vi "Statistics.vi"() -> ()   [LabVIEW 2023]
uses:
  <vilib>/Analysis/NI_AALBase.lvlib
panel:
  out "Variance My":dbl[](array[numeric])
  out "STD":dbl[](array[numeric])
  out "Average in row":u64[](array[numeric]) format="%-2.0f"
  out "Deviation by row":i64[][](array[numeric]) format="%.1f"
  out "Max in row":i32[](array[numeric])
  out "Min in row":i32[](array[numeric])
  out "Mean == Average":u64[](array[numeric])
  out "Variance":u64[](array[numeric])
  out "Std Deviation":dbl[](array[numeric]) format="%.4f"
  out "Mean":u64[](array[numeric])
  out "2D Double Array":i32[][](array[numeric])
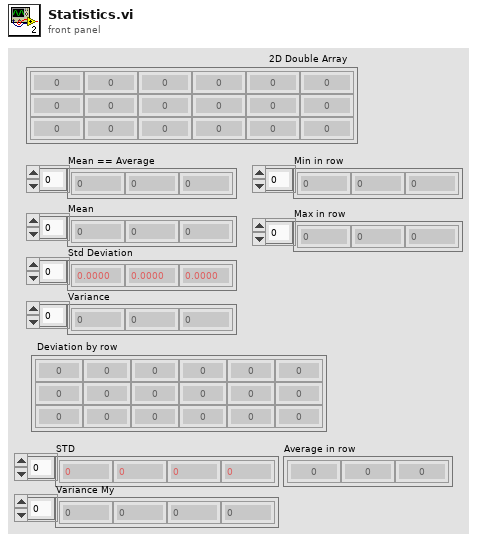
[diagram p1: front panel]
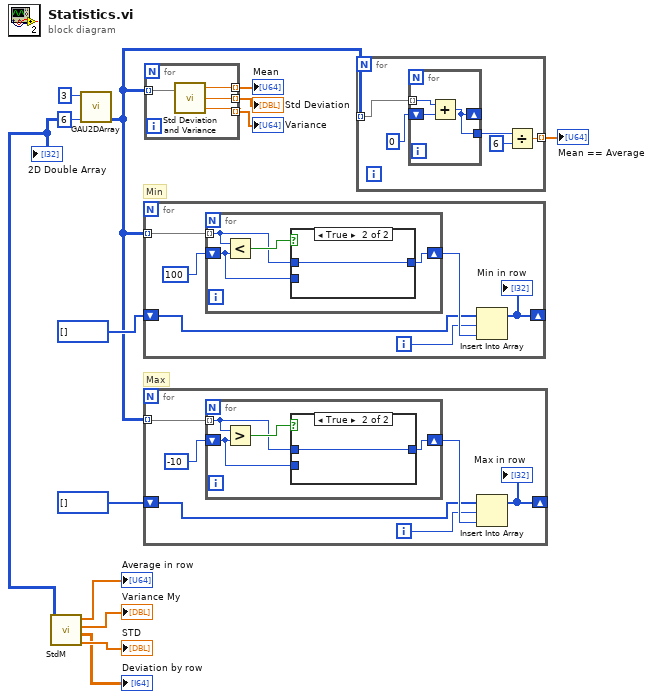
[diagram p0: block diagram]
diagram:
  # "Max"
  # "Min"
  n1 = call "GAU2DArray.vi"("Colums"=6, "Rows"=3) -> ("2D Double Array"=w5:i32[][])  [unwired: 7 in, 2 out]
  "2D Double Array" <- w5
  n2 = call "StdM.vi"("2D"=w5) -> ("My std"=→"STD":dbl[], "[Xi-X]"=→"Deviation by row":dbl[][], "Xi - X"=→"Variance My":dbl[], "Mean"=→"Average in row":dbl[])  [unwired: 6 in, 1 out]
  n3 = for {
    tunnel: w5 -> [w19] mode=indexing
    shift-right: [w15] -> _
    shift-left: i32[] [] -> [w14]
    i -> [w16]
    n4 = for {
      tunnel: w19 -> [w22] mode=indexing
      shift-right: [w21] -> w17
      shift-left: 100 ("element") -> [w20]
      n5 = Less?(x=w22, y=w20) -> (x < y?=w23:bool)
      n6 = case shown="True" w23 {
        tunnel: w22 -> [_ w25]
        tunnel: [w24 w25] -> w21
        tunnel: w20 -> [w24 _]
        frame False {
        }
        frame True {
        }
      }
    }
    n7 = Insert Into Array(array=w14, index=w16, new element=w17) -> (w15:i32[])
    "Min in row" <- w15
  }
  n8 = for {
    tunnel: w5 -> [w31] mode=indexing
    shift-right: [w27] -> _
    shift-left: i32[] [] -> [w26]
    i -> [w28]
    n9 = for {
      tunnel: w31 -> [w34] mode=indexing
      shift-right: [w33] -> w29
      shift-left: -10 ("element") -> [w32]
      n10 = Greater?(x=w34, y=w32) -> (0:w35:bool)
      n11 = case shown="True" w35 {
        tunnel: w34 -> [_ w37]
        tunnel: [w36 w37] -> w33
        tunnel: w32 -> [w36 _]
        frame False {
        }
        frame True {
        }
      }
    }
    n12 = Insert Into Array(array=w26, index=w28, new element=w29) -> (w27:i32[])
    "Max in row" <- w27
  }
  n13 = for {
    tunnel: w5 -> [w41] mode=indexing
    tunnel: [w40] -> w12 mode=indexing
    tunnel: [w39] -> w11 mode=indexing
    tunnel: [w38] -> w10 mode=indexing
    n14 = call <vilib>:"Std Deviation and Variance.vi"("X"=w41) -> ("mean"=w40:dbl, "standard deviation"=w39:dbl, "variance"=w38:dbl)  [unwired: 1 in]
  }
  "Mean" <- w12
  "Std Deviation" <- w11
  "Variance" <- w10
  n15 = for {
    tunnel: w5 -> [w46] mode=indexing
    tunnel: [w42] -> w8 mode=indexing
    n16 = for {
      tunnel: w46 -> [w49] mode=indexing
      shift-right: [w47] -> _
      shift-left: 0 -> [w48]
      tunnel: [w47] -> w44
      n17 = Add(x=w49, y=w48) -> (x+y=w47:i32)
    }
    n18 = Divide(x=w44, y=6) -> (x/y=w42:dbl)
  }
  "Mean == Average" <- w8
